vi "save_volume_set.vi"(8 "error in":errorcluster, 10 "matched set":set{cluster{"CLZ id":i32, "CV id":i32}}(c389), 11 "banary folder":path) -> (0 "error out":errorcluster)   [LabVIEW 2024, in "CLZ_to_ComicVine.lvlib"]
uses:
  CLZ_to_ComicVine.lvlib
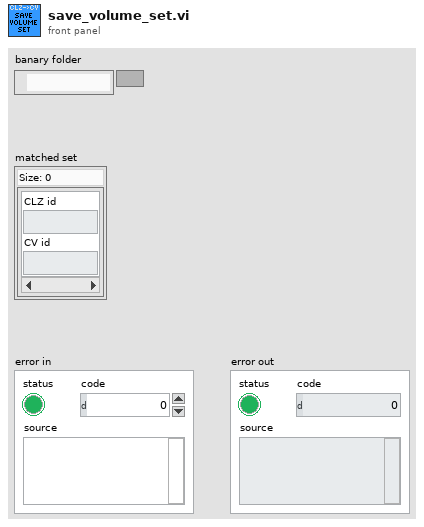
[diagram p1: front panel]
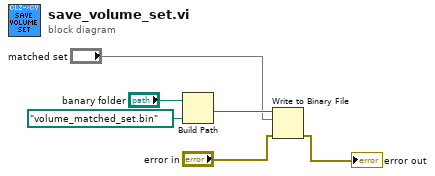
[diagram p0: block diagram]
diagram:
  n1 = Build Path(base path="banary folder", name or relative path=path "volume_matched_set.bin") -> (appended path=w4:path)
  n2 = Write to Binary File(file (use dialog)=w4, data="matched set", error in="error in") -> (error out=→"error out":errorcluster)  [unwired: 3 in, 2 out]
